vi "标样核查.vi"() -> ()   [LabVIEW 2016, in "斯坦道多参数.lvlib"]
panel:
  out "运行状态":u16(ring) items=["空闲", "水样测试", "标样核查"]
  out "seconds since 1Jan1904":timestamp
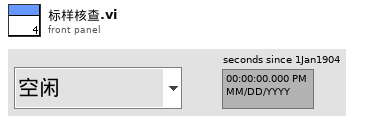
[diagram p1: front panel]
types:
  T1 = cluster{"ph":bool, "DO":bool, "Cond":bool, "Turb":bool, "叶绿素a":bool, "藻密度":bool, "ORP":bool, "cod":bool, "DO2":bool}
  T2 = cluster{"运行模式":enum16{"维护模式", "常规模式", "应急模式", "质控模式"}, "24H周期设置":bool[]}
  T3 = typedef "集成多参数单参数字段定义.ctl" = cluster{"时间":timestamp, "测量模式":string, "数据类型":string, "检测值":sgl, "单位":string, "数据标识":string, "信号值":sgl, "标样参考值":sgl, "因子编码":string, "探头温度":sgl, "LastTime":timestamp}
  T4 = typedef "LVDateTimeRec.ctl" = cluster{"秒数的小数部分":dbl, "秒":i32, "分":i32, "时":i32, "日":i32, "月":i32, "年":i32, "天数（周）":i32, "天数（年）":i32, "DST":i32}
  T5 = cluster{"数据保存间隔":dbl, "保存组数":dbl, "水温标样值":dbl, "pH标样值":dbl, "溶解氧标样值":dbl, "电导率标样值":dbl, "浊度标样值":dbl, "叶绿素a标样值":dbl, "藻密度标样值":dbl, "pH启用":bool, "溶解氧启用":bool, "电导率启用":bool, "浊度启用":bool, "叶绿素a启用":bool, "藻密度启用":bool}
  T6 = cluster{"温度测量值":sgl, "测量值":sgl, "温度偏移修正值":sgl, "信号值":sgl, "数据标识":string}
  T7 = cluster{"温度测量值":sgl, "DO%":sgl, "DOmg/L":sgl, "温度偏移修正值":sgl, "数据标识mg/L":string, "数据标识%":string}
  T8 = cluster{"CH":u16, "监测值":dbl, "信号值":sgl, "数据标识":string}
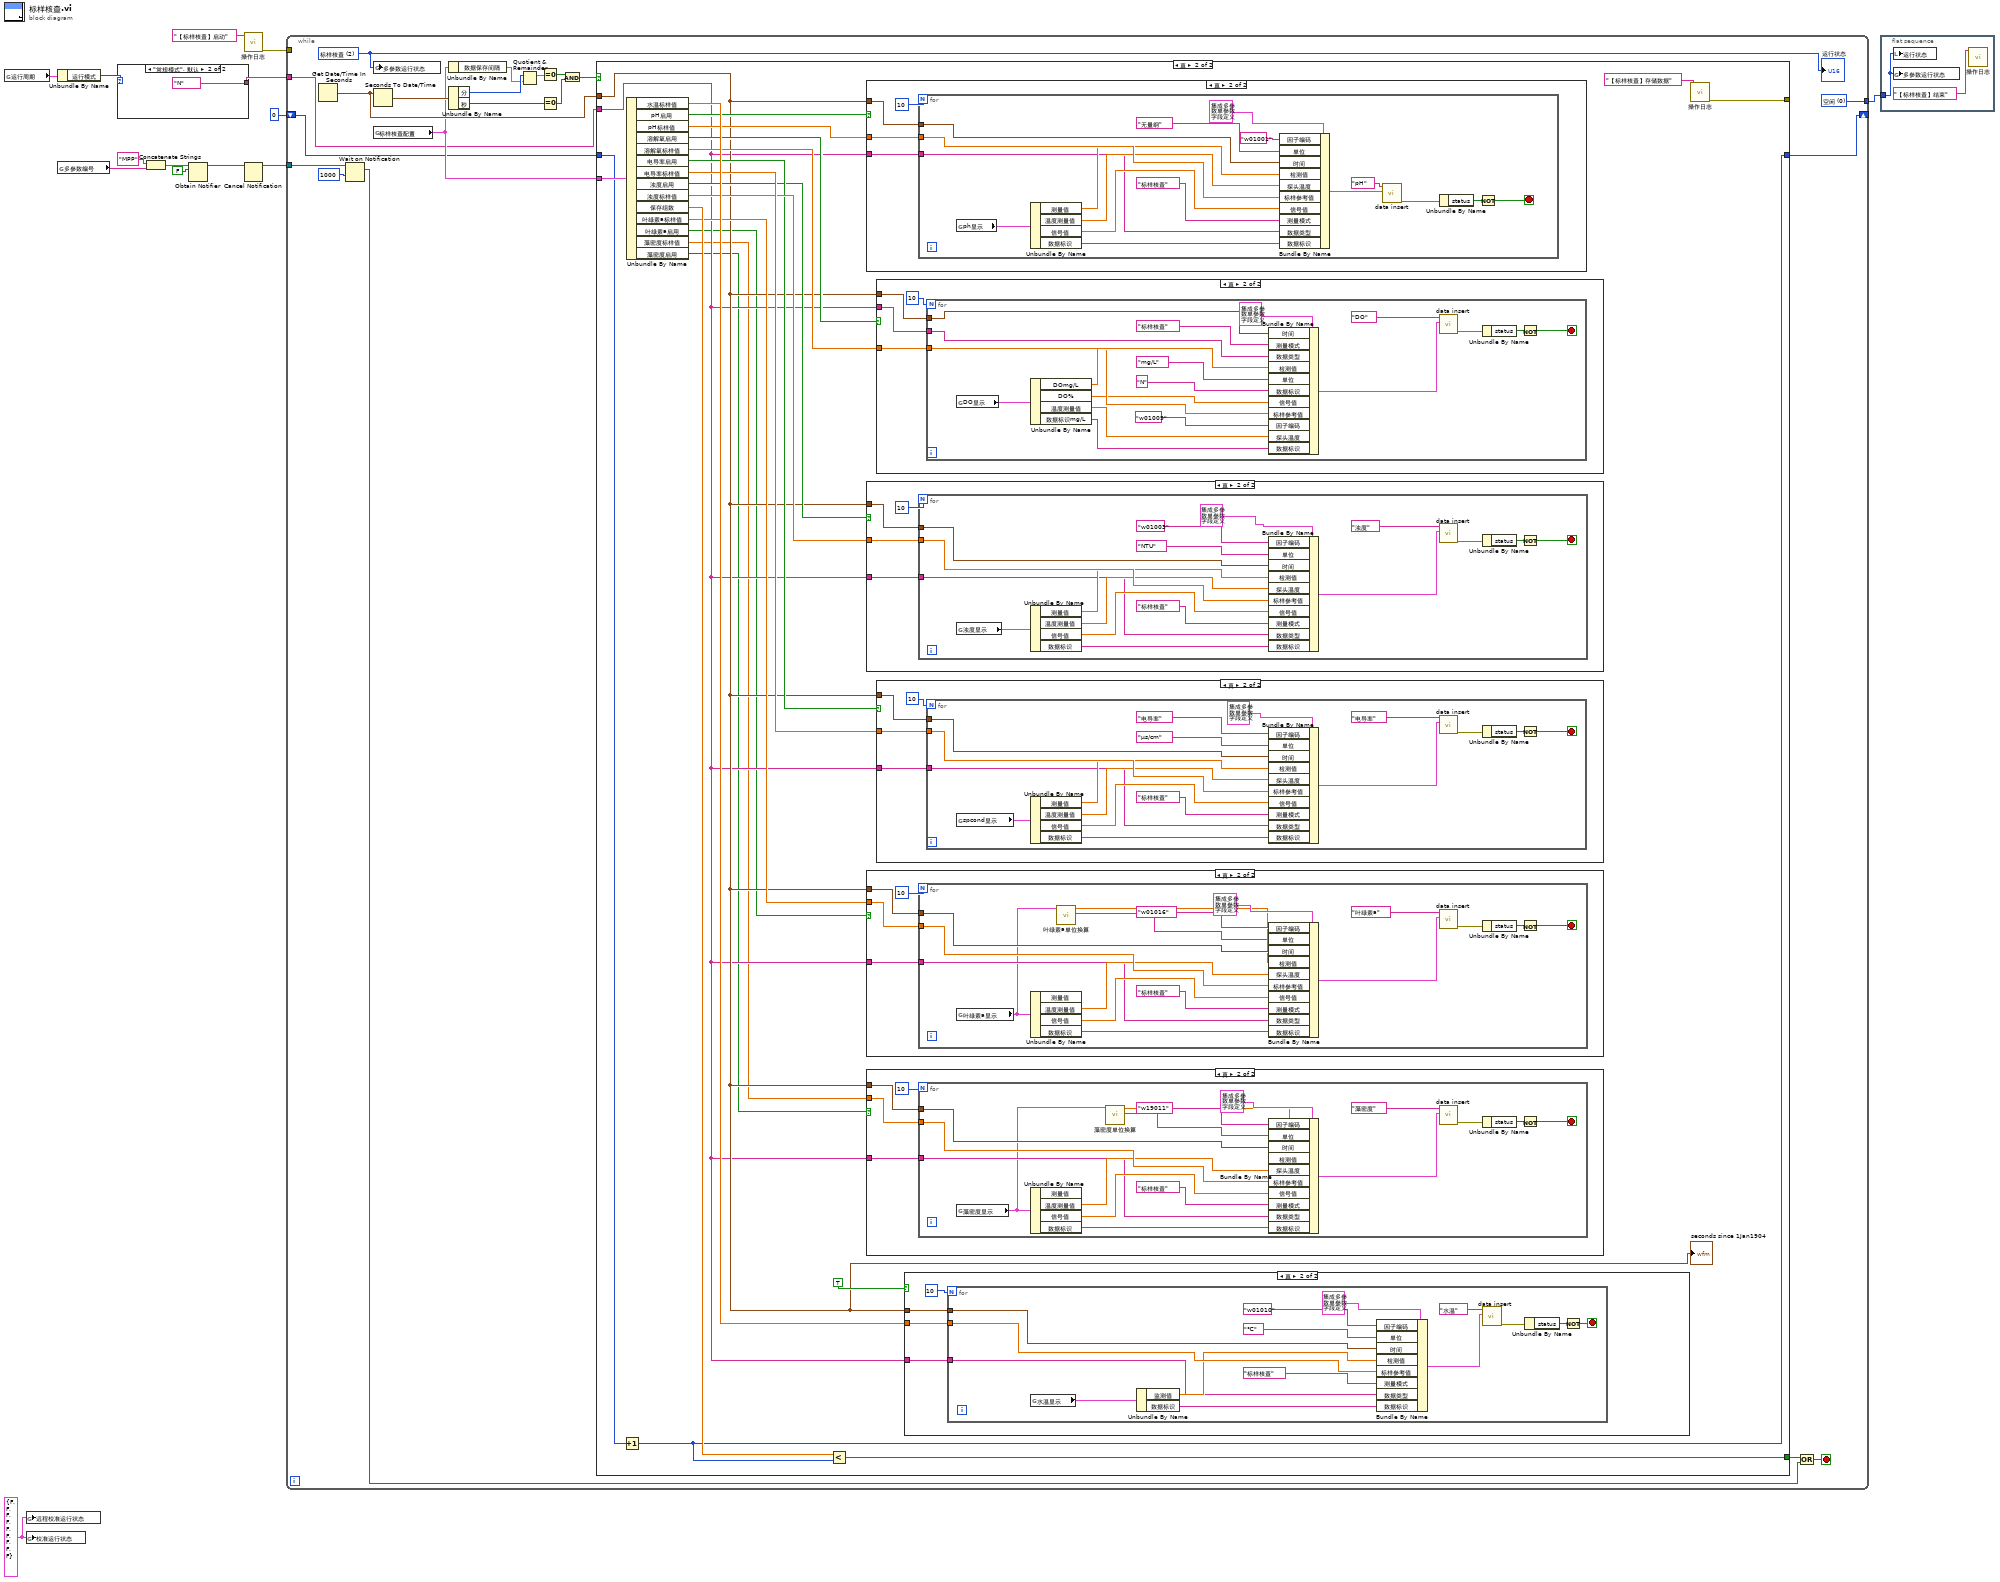
[diagram p0: block diagram]
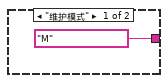
[diagram p2: hidden frame]
diagram:
  w4 = T1 {"ph"=FALSE, "DO"=FALSE, "Cond"=FALSE, "Turb"=FALSE, "叶绿素a"=FALSE, "藻密度"=FALSE, "ORP"=FALSE, "cod"=FALSE, "DO2"=FALSE} ("远程校准运行状态")
  n1 = global read "断电保存变量.vi" "运行周期"() -> (w2:T2)
  n2 = global write "多参数全局变量.vi" "远程校准运行状态"(w4) -> ()
  n3 = global write "多参数全局变量.vi" "校准运行状态"(w4) -> ()
  n4 = Unbundle By Name(w2) -> ("运行模式"=w1:enum16{"维护模式", "常规模式", "应急模式", "质控模式"})
  n5 = global read "多参数全局变量.vi" "多参数编号"() -> (w8:string)
  n6 = case shown="\"常规模式\", 默认" w1 {
    tunnel: ["M" ("数据标记表") "N" ("数据标记表")] -> w3
    frame "维护模式" {
    }
    frame "常规模式", Default {
    }
  }
  n7 = Concatenate Strings("MPP" ("名称（未命名）"), w8) -> (w9:string)
  n8 = Obtain Notifier(name (unnamed)=w9, notification data type=FALSE) -> (notifier out=w12:refnum<notifier>)  [unwired: 2 in, 2 out]
  n9 = call "操作日志.vi"("日志信息"="【标样核查】启动") -> ("error out"=w6:errorcluster)  [unwired: 10 in]
  n10 = Cancel Notification(0:w12) -> (8:w11:refnum<notifier>)  [unwired: 1 in, 2 out]
  n11 = while {
    tunnel: [w27] -> w10
    tunnel: w11 -> [w26]
    tunnel: w6 -> [_]
    shift-right: [w20] -> _
    shift-left: 0 -> [w21]
    tunnel: w3 -> [w17]
    stop <- w19 stop-if-true
    w27 = u16 0 items=["空闲", "水样测试", "标样核查"] ("多参数运行状态")
    w23 = u16 2 items=["空闲", "水样测试", "标样核查"] ("多参数运行状态")
    n12 = Get Date/Time In Seconds() -> (seconds since 1Jan1904=w28:timestamp)
    n13 = Wait on Notification(notifier=w26, timeout in ms (-1)=1000 ("超时毫秒(-1)")) -> (notification=w24:bool)  [unwired: 2 in, 3 out]
    n14 = global write "多参数全局变量.vi" "多参数运行状态"(w23) -> ()
    n15 = Seconds To Date/Time(time stamp (now)=w28) -> (date time rec=w36:T4)  [unwired: 1 in]
    n16 = global read "断电保存变量.vi" "标样核查配置"() -> (w22:T5)
    n17 = Unbundle By Name(w22) -> ("数据保存间隔"=w31:dbl)
    n18 = Unbundle By Name(w36) -> ("分"=w32:i32, "秒"=w35:i32)
    n19 = Quotient & Remainder(x=w32, y=w31) -> (x-y*floor(x/y)=w30:dbl)  [unwired: 1 out]
    n20 = Equal To 0?(x=w30) -> (x = 0?=w29:bool)
    n21 = Equal To 0?(x=w35) -> (x = 0?=w34:bool)
    n22 = And(x=w29, y=w34) -> (x .and. y?=w33:bool)
    n23 = case shown="真" w33 {
      tunnel: w22 -> [_ w60]
      tunnel: w28 -> [_ w42]
      tunnel: [_ w53] -> _
      tunnel: w21 -> [w37 w47]
      tunnel: [w37 w45] -> w20
      tunnel: [_ w44] -> w18
      tunnel: w17 -> [_ w41]
      frame False {
      }
      frame True {
        n24 = Increment(x=w47) -> (x+1=w45:i32)
        n25 = Unbundle By Name(w60) -> ("水温标样值"=w59:dbl, "pH启用"=w52:bool, "pH标样值"=w58:dbl, "溶解氧启用"=w50:bool, "溶解氧标样值"=w57:dbl, "电导率启用"=w49:bool, "电导率标样值"=w56:dbl, "浊度启用"=w48:bool, "浊度标样值"=w55:dbl, "保存组数"=w46:dbl, "叶绿素a标样值"=w43:dbl, "叶绿素a启用"=w38:bool, "藻密度标样值"=w40:dbl, "藻密度启用"=w39:bool)
        n26 = Less?(x=w46, y=w45) -> (x < y?=w44:bool)
        n27 = case shown="真" w52 {
          tunnel: w58 -> [_ w170]
          tunnel: w42 -> [_ w168]
          tunnel: w41 -> [_ w167]
          frame False {
          }
          frame True {
            n28 = for {
              N: 10 -> [_]
              tunnel: w170 -> [w184]
              tunnel: w168 -> [w177]
              tunnel: w167 -> [w172]
              stop <- w178 stop-if-true
              n29 = global read "多参数全局变量.vi" "ph显示"() -> (w183:T6)
              n30 = Unbundle By Name(w183) -> ("测量值"=w182:sgl, "温度测量值"=w181:sgl, "信号值"=w175:sgl, "数据标识"=w173:string)
              n31 = Bundle By Name(cluster=T3 {"时间"=timestamp(0 s since 1904-01-01), "测量模式"="水样测试", "数据类型"="N", "检测值"=0.0, "单位"="mg/L", "数据标识"="N", "信号值"=0.0, "标样参考值"=0.0, "因子编码"="", "探头温度"=0.0, "LastTime"=timestamp(0 s since 1904-01-01)} ("data"), "因子编码"="w01001", "单位"="无量纲", "时间"=w177, "检测值"=w182, "探头温度"=w181, "标样参考值"=w184, "信号值"=w175, "测量模式"="标样核查", "数据类型"=w172, "数据标识"=w173) -> (w176:T3)
              n32 = call "data insert.vi"("data"=w176, "table in"="pH" ("table输入")) -> ("error out"=w180:errorcluster)  [unwired: 9 in]
              n33 = Unbundle By Name(w180) -> ("status"=w179:bool)
              n34 = Not(x=w179) -> (.not. x?=w178:bool)
            }
          }
        }
        n35 = case shown="真" w48 {
          tunnel: w55 -> [_ w106]
          tunnel: w42 -> [_ w104]
          tunnel: w41 -> [_ w103]
          frame False {
          }
          frame True {
            n36 = for {
              N: 10 -> [_]
              tunnel: w106 -> [w119]
              tunnel: w104 -> [w112]
              tunnel: w103 -> [w108]
              stop <- w113 stop-if-true
              n37 = global read "多参数全局变量.vi" "浊度显示"() -> (w118:T6)
              n38 = Unbundle By Name(w118) -> ("测量值"=w117:sgl, "温度测量值"=w116:sgl, "信号值"=w111:sgl, "数据标识"=w109:string)
              n39 = Bundle By Name(cluster=T3 {"时间"=timestamp(0 s since 1904-01-01), "测量模式"="水样测试", "数据类型"="N", "检测值"=0.0, "单位"="mg/L", "数据标识"="N", "信号值"=0.0, "标样参考值"=0.0, "因子编码"="", "探头温度"=0.0, "LastTime"=timestamp(0 s since 1904-01-01)} ("data"), "因子编码"="w01003", "单位"="NTU", "时间"=w112, "检测值"=w117, "探头温度"=w116, "标样参考值"=w119, "信号值"=w111, "测量模式"="标样核查", "数据类型"=w108, "数据标识"=w109) -> (w122:T3)
              n40 = call "data insert.vi"("data"=w122, "table in"="浊度" ("table输入")) -> ("error out"=w115:errorcluster)  [unwired: 9 in]
              n41 = Unbundle By Name(w115) -> ("status"=w114:bool)
              n42 = Not(x=w114) -> (.not. x?=w113:bool)
            }
          }
        }
        n43 = case shown="真" w38 {
          tunnel: w43 -> [_ w85]
          tunnel: w42 -> [_ w83]
          tunnel: w41 -> [_ w82]
          frame False {
          }
          frame True {
            n44 = for {
              N: 10 -> [_]
              tunnel: w85 -> [w99]
              tunnel: w83 -> [w94]
              tunnel: w82 -> [w90]
              stop <- w95 stop-if-true
              n45 = global read "多参数全局变量.vi" "叶绿素a显示"() -> (w88:T6)
              n46 = Unbundle By Name(w88) -> ("温度测量值"=w98:sgl, "信号值"=w93:sgl, "数据标识"=w91:string)  [unwired: 1 out]
              n47 = call "叶绿素a单位换算.vi"("叶绿素a显示"=w88) -> ("检测值1.单位"=w86:string, "测量值"=w87:sgl)  [unwired: 8 in, 1 out]
              n48 = Bundle By Name(cluster=T3 {"时间"=timestamp(0 s since 1904-01-01), "测量模式"="水样测试", "数据类型"="N", "检测值"=0.0, "单位"="mg/L", "数据标识"="N", "信号值"=0.0, "标样参考值"=0.0, "因子编码"="", "探头温度"=0.0, "LastTime"=timestamp(0 s since 1904-01-01)} ("data"), "因子编码"="w01016", "单位"=w86, "时间"=w94, "检测值"=w87, "探头温度"=w98, "标样参考值"=w99, "信号值"=w93, "测量模式"="标样核查", "数据类型"=w90, "数据标识"=w91) -> (w102:T3)
              n49 = call "data insert.vi"("data"=w102, "table in"="叶绿素a" ("table输入")) -> ("error out"=w97:errorcluster)  [unwired: 9 in]
              n50 = Unbundle By Name(w97) -> ("status"=w96:bool)
              n51 = Not(x=w96) -> (.not. x?=w95:bool)
            }
          }
        }
        n52 = case shown="真" w39 {
          tunnel: w40 -> [_ w64]
          tunnel: w42 -> [_ w62]
          tunnel: w41 -> [_ w61]
          frame False {
          }
          frame True {
            n53 = for {
              N: 10 -> [_]
              tunnel: w64 -> [w78]
              tunnel: w62 -> [w73]
              tunnel: w61 -> [w69]
              stop <- w74 stop-if-true
              n54 = global read "多参数全局变量.vi" "藻密度显示"() -> (w67:T6)
              n55 = Unbundle By Name(w67) -> ("温度测量值"=w77:sgl, "信号值"=w72:sgl, "数据标识"=w70:string)  [unwired: 1 out]
              n56 = call "藻密度单位换算.vi"("藻密度显示"=w67) -> ("检测值1.单位"=w66:string, "测量值"=w65:sgl)  [unwired: 8 in, 1 out]
              n57 = Bundle By Name(cluster=T3 {"时间"=timestamp(0 s since 1904-01-01), "测量模式"="水样测试", "数据类型"="N", "检测值"=0.0, "单位"="mg/L", "数据标识"="N", "信号值"=0.0, "标样参考值"=0.0, "因子编码"="", "探头温度"=0.0, "LastTime"=timestamp(0 s since 1904-01-01)} ("data"), "因子编码"="w19011", "单位"=w66, "时间"=w73, "检测值"=w65, "探头温度"=w77, "标样参考值"=w78, "信号值"=w72, "测量模式"="标样核查", "数据类型"=w69, "数据标识"=w70) -> (w81:T3)
              n58 = call "data insert.vi"("data"=w81, "table in"="藻密度" ("table输入")) -> ("error out"=w76:errorcluster)  [unwired: 9 in]
              n59 = Unbundle By Name(w76) -> ("status"=w75:bool)
              n60 = Not(x=w75) -> (.not. x?=w74:bool)
            }
          }
        }
        n61 = case shown="真" w50 {
          tunnel: w57 -> [_ w148]
          tunnel: w42 -> [_ w146]
          tunnel: w41 -> [_ w145]
          frame False {
          }
          frame True {
            n62 = for {
              N: 10 -> [_]
              tunnel: w148 -> [w156]
              tunnel: w146 -> [w161]
              tunnel: w145 -> [w150]
              stop <- w164 stop-if-true
              n63 = global read "多参数全局变量.vi" "DO显示"() -> (w166:T7)
              n64 = Unbundle By Name(w166) -> ("DOmg/L"=w159:sgl, "DO%"=w153:sgl, "温度测量值"=w152:sgl, "数据标识mg/L"=w151:string)
              n65 = Bundle By Name(cluster=T3 {"时间"=timestamp(0 s since 1904-01-01), "测量模式"="水样测试", "数据类型"="N", "检测值"=0.0, "单位"="mg/L", "数据标识"="N", "信号值"=0.0, "标样参考值"=0.0, "因子编码"="", "探头温度"=0.0, "LastTime"=timestamp(0 s since 1904-01-01)} ("data"), "时间"=w161, "测量模式"="标样核查", "数据类型"=w150, "检测值"=w159, "单位"="mg/L", "数据标识"="N" ("水样数据标识"), "信号值"=w153, "标样参考值"=w156, "因子编码"="w01009", "探头温度"=w152, "数据标识"=w151) -> (w162:T3)
              n66 = call "data insert.vi"("data"=w162, "table in"="DO") -> ("error out"=w154:errorcluster)  [unwired: 9 in]
              n67 = Unbundle By Name(w154) -> ("status"=w165:bool)
              n68 = Not(x=w165) -> (.not. x?=w164:bool)
            }
          }
        }
        n69 = case shown="真" w49 {
          tunnel: w56 -> [_ w127]
          tunnel: w42 -> [_ w125]
          tunnel: w41 -> [_ w124]
          frame False {
          }
          frame True {
            n70 = for {
              N: 10 -> [_]
              tunnel: w127 -> [w141]
              tunnel: w125 -> [w134]
              tunnel: w124 -> [w129]
              stop <- w135 stop-if-true
              n71 = global read "多参数全局变量.vi" "spcond显示"() -> (w140:T6)
              n72 = Unbundle By Name(w140) -> ("测量值"=w139:sgl, "温度测量值"=w138:sgl, "信号值"=w132:sgl, "数据标识"=w130:string)
              n73 = Bundle By Name(cluster=T3 {"时间"=timestamp(0 s since 1904-01-01), "测量模式"="水样测试", "数据类型"="N", "检测值"=0.0, "单位"="mg/L", "数据标识"="N", "信号值"=0.0, "标样参考值"=0.0, "因子编码"="", "探头温度"=0.0, "LastTime"=timestamp(0 s since 1904-01-01)} ("data"), "因子编码"="电导率", "单位"="μs/cm", "时间"=w134, "检测值"=w139, "探头温度"=w138, "标样参考值"=w141, "信号值"=w132, "测量模式"="标样核查", "数据类型"=w129, "数据标识"=w130) -> (w144:T3)
              n74 = call "data insert.vi"("data"=w144, "table in"="电导率" ("table输入")) -> ("error out"=w137:errorcluster)  [unwired: 9 in]
              n75 = Unbundle By Name(w137) -> ("status"=w136:bool)
              n76 = Not(x=w136) -> (.not. x?=w135:bool)
            }
          }
        }
        n77 = case shown="真" TRUE {
          tunnel: w59 -> [_ w191]
          tunnel: w42 -> [_ w190]
          tunnel: w41 -> [_ w188]
          frame False {
          }
          frame True {
            n78 = for {
              N: 10 -> [_]
              tunnel: w191 -> [w202]
              tunnel: w190 -> [w199]
              tunnel: w188 -> [w193]
              stop <- w196 stop-if-true
              n79 = global read "多参数全局变量.vi" "水温显示"() -> (w201:T8)
              n80 = Unbundle By Name(w201) -> ("监测值"=w200:dbl, "数据标识"=w194:string)
              n81 = Bundle By Name(cluster=T3 {"时间"=timestamp(0 s since 1904-01-01), "测量模式"="水样测试", "数据类型"="N", "检测值"=0.0, "单位"="mg/L", "数据标识"="N", "信号值"=0.0, "标样参考值"=0.0, "因子编码"="", "探头温度"=0.0, "LastTime"=timestamp(0 s since 1904-01-01)} ("data"), "因子编码"="w01010", "单位"="℃", "时间"=w199, "检测值"=w200, "标样参考值"=w202, "测量模式"="标样核查", "数据类型"=w193, "数据标识"=w194) -> (w205:T3)
              n82 = call "data insert.vi"("data"=w205, "table in"="水温" ("table输入")) -> ("error out"=w198:errorcluster)  [unwired: 9 in]
              n83 = Unbundle By Name(w198) -> ("status"=w197:bool)
              n84 = Not(x=w197) -> (.not. x?=w196:bool)
            }
          }
        }
        n85 = call "操作日志.vi"("日志信息"="【标样核查】存储数据") -> ("error out"=w53:errorcluster)  [unwired: 10 in]
        "seconds since 1Jan1904" <- w42
      }
    }
    n86 = Or(x=w18, y=w24) -> (x .or. y?=w19:bool)
    "运行状态" <- w23
  }
  n87 = flat-sequence {
    tunnel: w10 -> [w208]
    frame #0 {
      n88 = local write "运行状态"(w208) -> ()
      n89 = global write "多参数全局变量.vi" "多参数运行状态"(w208) -> ()
      n90 = call "操作日志.vi"("日志信息"="【标样核查】结束") -> ()  [unwired: 10 in, 1 out]
    }
  }
